vi "Autocorrelation_ph.vi"(0 "X":dbl[](array[numeric]) format="%.2f", 3 "Autocorrelation of X":dbl[](array[numeric]) format="%.4f", 4 "Block No":i32=1) -> (6 "Autocorrelation of X":dbl[](array[numeric]) format="%.4f")   [LabVIEW 2010]
uses:
  <vilib>/Analysis/2dsp.llb/1D Auto Correlation (DBL).vi
  <vilib>/Analysis/NI_AALBase.lvlib
  <vilib>/Analysis/NI_AALPro.lvlib
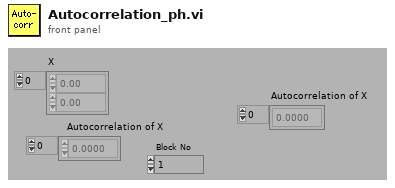
[diagram p1: front panel]
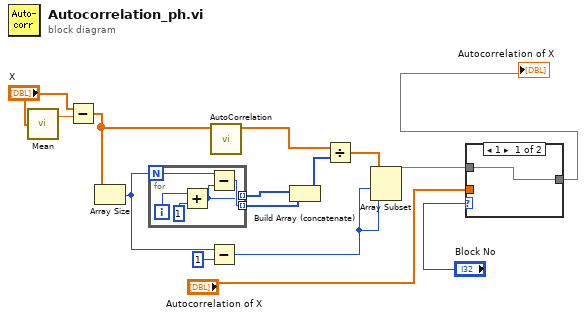
[diagram p0: block diagram]
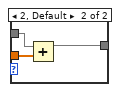
[diagram p2: hidden frame]
diagram:
  n1 = call <vilib>:"Mean.vi"("X"="X") -> ("mean"=w7:dbl)  [unwired: 1 out]
  n2 = Subtract(x="X", y=w7) -> (x-y=w5:dbl[])
  n3 = Array Size(array=w5) -> (size(s)=w8:i32)
  n4 = for {
    N: w8 -> [w20]
    tunnel: [w17] -> w13 mode=indexing
    tunnel: [w18] -> w15 mode=indexing
    i -> [w19]
    n5 = Add(x=w19, y=1) -> (x+y=w17:i32)
    n6 = Subtract(x=w20, y=w17) -> (x-y=w18:i32)
  }
  n7 = Subtract(x=w8, y=1) -> (x-y=w9:i32)
  n8 = call-poly <vilib>:"AutoCorrelation.vi"("X"=w5) -> ("Rxx"=w14:dbl[])  [unwired: 1 in, 9 out]
  n9 = Build Array (concatenate)(w13, w15) -> (w12:i32[])
  n10 = Divide(x=w14, y=w12) -> (x/y=w11:dbl[])
  n11 = Array Subset(array=w11, index=w9, length=w9) -> (w4:dbl[])
  n12 = case shown="1" "Block No" {
    tunnel: [w21 w24] -> w2
    tunnel: w4 -> [w21 w23]
    tunnel: "Autocorrelation of X" -> [_ w22]
    frame 1 {
    }
    frame 2, Default {
      n13 = Add(x=w23, y=w22) -> (x+y=w24:dbl[])
    }
  }
  "Autocorrelation of X" <- w2
